vi "Get Instrument Path.vi"(8 "error in":errorcluster, 11 "instrument_type_id":string) -> (0 "error out":errorcluster, 3 "Instrument Path":path)   [LabVIEW 2021, in "Get Pin Information.lvlib"]
uses:
  Get Pin Information.lvlib
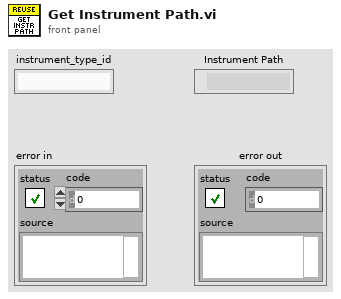
[diagram p1: front panel]
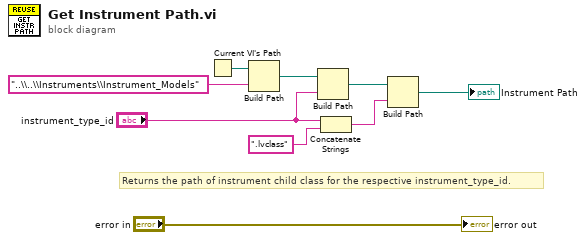
[diagram p0: block diagram]
diagram:
  # "Returns the path of instrument child class for the respective instrument_type_id."
  n1 = Current VI's Path() -> (path=w7:path)
  n2 = Build Path(base path=w7, name or relative path="..\\..\\Instruments\\Instrument_Models") -> (appended path=w4:path)
  n3 = Build Path(base path=w4, name or relative path="instrument_type_id") -> (appended path=w2:path)
  n4 = Concatenate Strings("instrument_type_id", ".lvclass" ("string")) -> (w9:string)
  n5 = Build Path(base path=w2, name or relative path=w9) -> (appended path=→"Instrument Path":path)
  "error out" <- "error in"
